vi "Make Test CAse.vi"(8 "error in (no error)":errorcluster) -> (0 "error out":errorcluster, 3 "LUnit Test Suite V2 out":refnum<class "LUnit Test Suite V2.lvclass">)   [LabVIEW 2020, in "Test Runner Test.lvclass"]
uses:
  Test Runner Test.lvclass
  LUnit Test Suite/LUnit Test Suite V2.lvclass
  Light Test Case Double/Light Test Case Double.lvclass
  C:/Git/astemes-lunit/source/Rewrite Project/LUnit Test Case/LUnit Test Case V2.lvclass
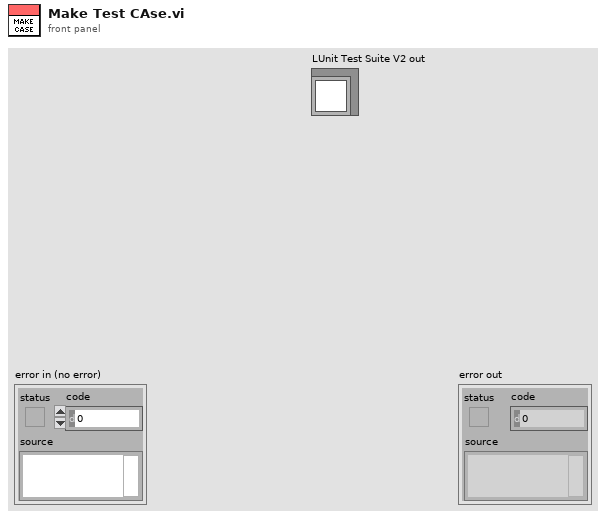
[diagram p1: front panel]
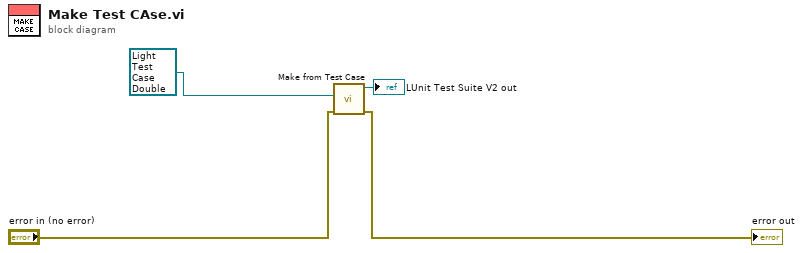
[diagram p0: block diagram]
diagram:
  n1 = call "Make from Test Case.vi"("error in (no error)"="error in (no error)", "LUnit Test Case"=refnum<class "Light Test Case Double.lvclass"> refnum ("Light Test Case Double.lvclass")) -> ("error out"=→"error out":errorcluster, "LUnit Test Suite V2 out"=→"LUnit Test Suite V2 out":refnum<class "LUnit Test Suite V2.lvclass">)  [unwired: 8 in]
